vi "Validate Endpoint Aliases Reference.vi"(8 "error in":errorcluster, 11 "endpoint aliases in":T1 format="%.0x") -> (0 "error out":errorcluster, 3 "endpoint aliases out":T1 format="%.0x")   [LabVIEW 2020, in "Routing and Faulting Scripting.lvlib"]
uses:
  Routing and Faulting Scripting.lvlib
  <vilib>/NI VeriStand/Custom Device API/Custom Device Item Ref.ctl
  Shared/Constants.vi
  Dependencies.llb/Routing and Faulting Shared.lvlib
  <vilib>/NI VeriStand/Custom Device API/Custom Device API.lvlib
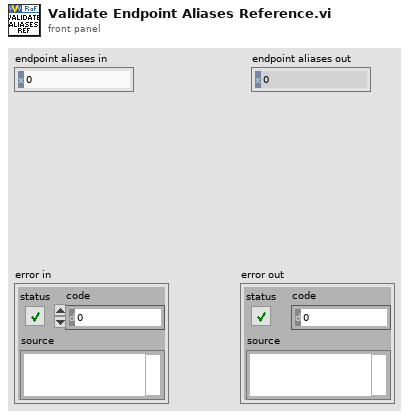
[diagram p1: front panel]
types:
  T1 = typedef "Custom Device API.lvlib/Custom Device Item Ref.ctl" = u64
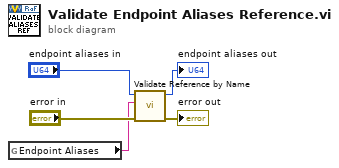
[diagram p0: block diagram]
diagram:
  n1 = global read "Constants.vi" "Endpoint Aliases"() -> (w1:string)
  n2 = call "Validate Reference by Name.vi"("error in"="error in", "name"=w1, "item in"="endpoint aliases in") -> ("error out"=→"error out":errorcluster, "item out"=→"endpoint aliases out":T1)  [unwired: 7 in]
